vi "220426_delta_cappture.vi"(3 "start Col.":i32, 4 "end Col.":i32, 5 "Rawdata pixmap":u8[][](array[numeric])=array40x561[22440 elements] caption="Input pixmap") -> (0 "TapN":dbl, 1 "moving Log(Y, X)":i32[][](array[numeric]), 2 "Total point":i32)   [LabVIEW 2016]
panel:
  out "progressLog":dbl[][](array[numeric])
  out "progress":dbl
  out "Δ":dbl
  out "point log":i32[](array[numeric])
  out "vertical":i32
  # "How to use : \nΔ = (vertical 40) / (23-22) ) = 40 \nΔ = (vertical 20) / (30-20) ) =  2 \nΔ = (vertical 35) / (23-20) ) = 11.67"
  # "Round (i / 11.67)\n  i  : prog. \n  0 : 0\n  1 : 0\n  4 : 0\n  5 : 1\n17 : 1\n18 : 2\n29 : 2\n30 : 3\n35 : 3"
  # "Δ ="
  # "="
  # "ー"
  # "progress = Round( i / Δ ) ="
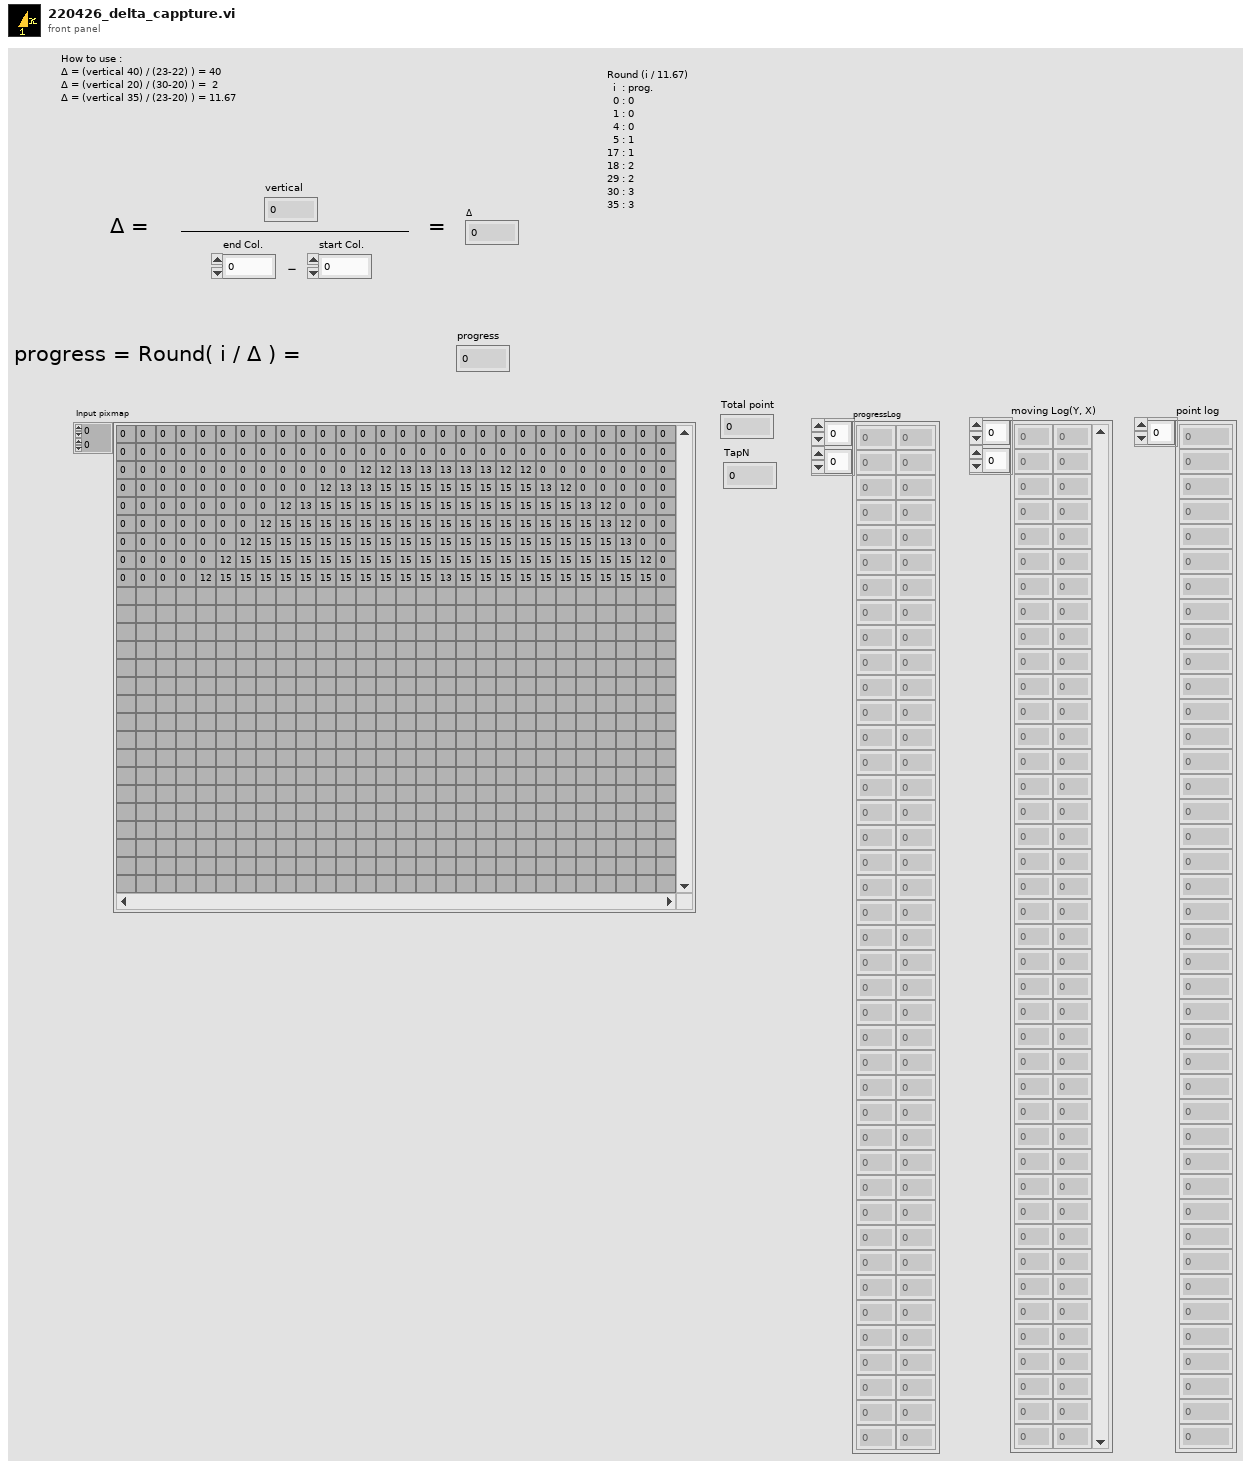
[diagram p1: front panel]
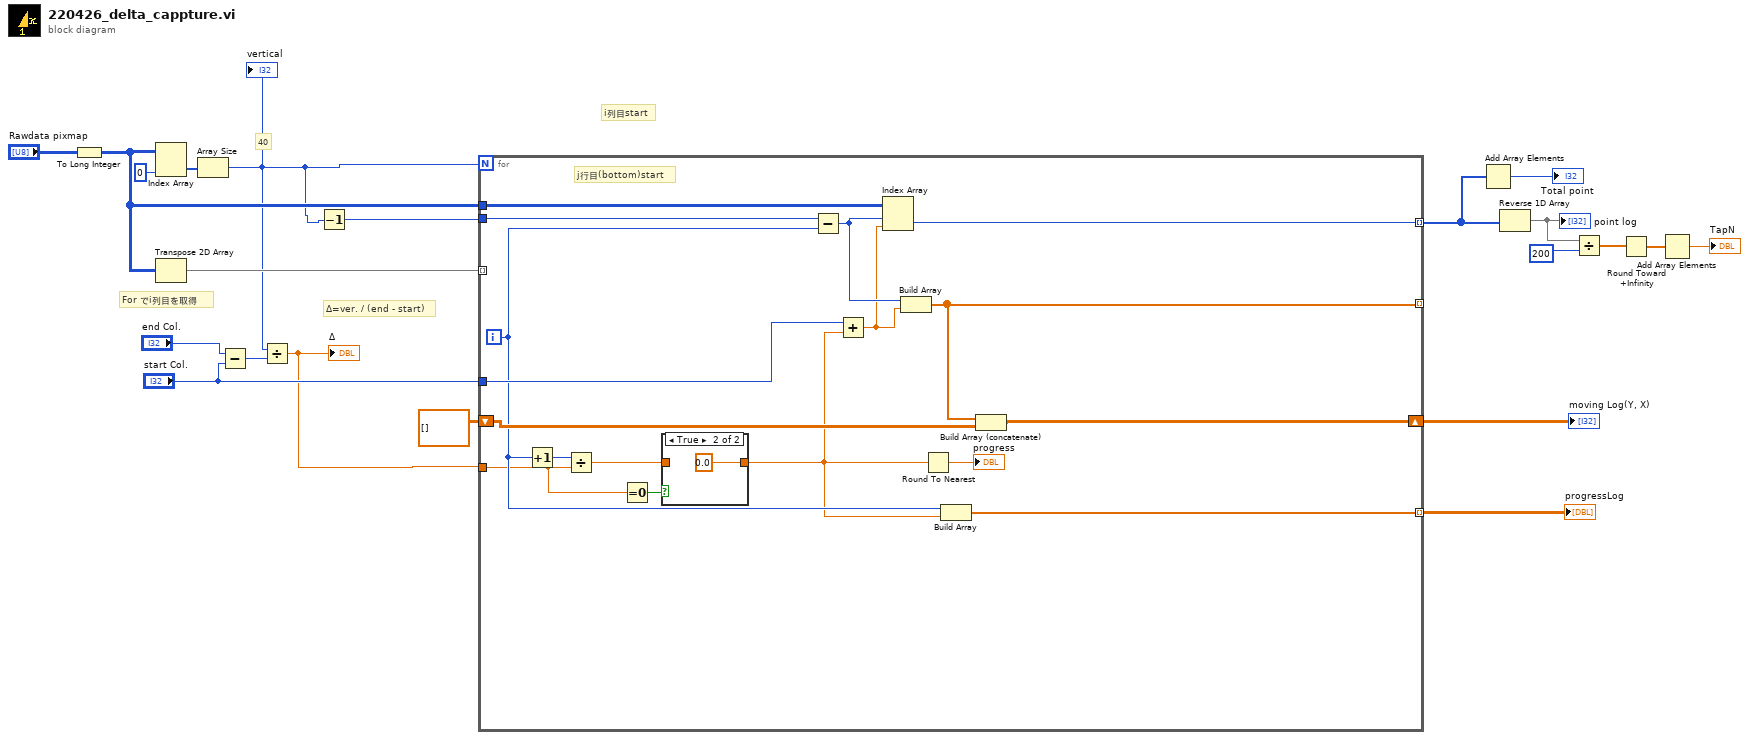
[diagram p0: block diagram]
diagram:
  # "Δ=ver. / (end - start)"
  # "i列目start"
  # "40"
  # "For でi列目を取得"
  n1 = To Long Integer(number="Rawdata pixmap") -> (32bit integer=w18:i32[][])
  n2 = Index Array(array=w18, index (col)=0 ("無効な指標 （列）")) -> (element=w19:i32[])  [unwired: 1 in]
  n3 = Transpose 2D Array(2D array=w18) -> (transposed array=w17:i32[][])
  n4 = Array Size(array=w19) -> (size(s)=w10:i32)
  "vertical" <- w10
  n5 = Subtract(x="end Col.", y="start Col.") -> (x-y=w2:i32)
  n6 = Divide(x=w10, y=w2) -> (x/y=w1:dbl)
  "Δ" <- w1
  n7 = Decrement(x=w10) -> (x-1=w15:i32)
  n8 = for {
    N: w10 -> [_]
    tunnel: w17 -> [_] mode=indexing
    tunnel: w15 -> [w37]
    tunnel: w18 -> [w38]
    tunnel: [w36] -> w8 mode=indexing
    tunnel: [w32] -> _ mode=indexing
    tunnel: "start Col." -> [w30]
    shift-right: [w33] -> w13
    shift-left: dbl[][] [] -> [w31]
    tunnel: w1 -> [w25]
    tunnel: [w29] -> w9 mode=indexing
    i -> [w27]
    # "j行目(bottom)start"
    n9 = Increment(x=w27) -> (x+1=w28:i32)
    n10 = Divide(x=w28, y=w25) -> (x/y=w24:dbl)
    n11 = Equal To 0?(x=w25) -> (x = 0?=w26:bool)
    n12 = case shown="True" w26 {
      tunnel: w24 -> [w39 _]
      tunnel: [w39 0.0] -> w22
      frame False {
      }
      frame True {
      }
    }
    n13 = Subtract(x=w37, y=w27) -> (x-y=w35:i32)
    n14 = Add(x=w30, y=w22) -> (x+y=w34:dbl)
    n15 = Index Array(array=w38, index (row)=w35, index (col)=w34) -> (element=w36:i32)
    n16 = Build Array(w35, w34) -> (w32:dbl[])
    n17 = Round To Nearest(number=w22) -> (nearest integer value=→"progress":dbl)
    n18 = Build Array(w27, w22) -> (w29:dbl[])
    n19 = Build Array (concatenate)(w32, w31) -> (w33:dbl[][])
  }
  "moving Log(Y, X)" <- w13
  "progressLog" <- w9
  n20 = Add Array Elements(numeric array=w8) -> (sum=→"Total point":i32)
  n21 = Reverse 1D Array(array=w8) -> (reversed array=w7:i32[])
  "point log" <- w7
  n22 = Divide(x=w7, y=200) -> (x/y=w5:dbl[])
  n23 = Round Toward +Infinity(x=w5) -> (ceil(x): smallest int >= x=w4:dbl[])
  n24 = Add Array Elements(numeric array=w4) -> (sum=→"TapN":dbl)
